vi "Planck-Curve-Sun-Earth.vi"() -> ()   [LabVIEW 2012]
panel:
  in  "Radius Sun (km)":dbl[unit]=696300.0
  in  "Distance Sun-Earth (km)":dbl[unit]=149600000.0
  out "Integral emittance (W m-2) 2":dbl[unit]=348.509952
  out "Integral emittance reaching Earth* (W m-2)":dbl[unit]=342.26526039686814
  out "Max emission (µm)":dbl=10.3525
  out "Max. emission (µm)":dbl=0.5016787815853236
  in  "Temperature of Earth (K)":dbl=280.0 step=10.0
  out "Planck Curves":T1(graph)=[{[{0.1, "Spectral emittance"=8.364960435276347e-211}, {0.19990000000000002, "Spectral emittance"=8.6959170545306e-101}, {0.2998, "Spectral emittance"=1.8099170209444927e-64}, {0.39970000000000006, "Spectral emittance"=1.7259097573278146e-46}, {0.49960000000000004, "Spectral emittance"=8.248773701500351e-36}, {0.5995, "Spectral emittance"=9.198523833864638e-29}, {0.6994, "Spectral emittance"=8.828454193587492e-24}, {0.7993, "Spectral emittance"=4.4031815212407465e-20}, {0.8992, "Spectral emittance"=3.0885678859060627e-17}, {0.9991, "Spectral emittance"=5.526298362014247e-15}, {1.099, "Spectral emittance"=3.679604984270012e-13}, {1.1989, "Spectral emittance"=1.1717326507920772e-11}, {1.2988000000000002, "Spectral emittance"=2.1218031119056521e-10}, {1.3987, "Spectral emittance"=2.4714773986706854e-09}, {1.4986000000000002, "Spectral emittance"=2.026296957778333e-08}, {1.5985, "Spectral emittance"=1.2507918319570943e-07}, {1.6984000000000001, "Spectral emittance"=6.119092116801698e-07}, {1.7983000000000002, "Spectral emittance"=2.4687793597519062e-06}, {1.8982, "Spectral emittance"=8.475417144153042e-06}, {1.9981000000000002, "Spectral emittance"=2.538389327407048e-05}, {2.098, "Spectral emittance"=6.767286542067558e-05}, {2.1979, "Spectral emittance"=0.00016325141397348066}, {2.2978, "Spectral emittance"=0.0003612038583115582}, {2.3977, "Spectral emittance"=0.0007412641406731495}, {2.4976000000000003, "Spectral emittance"=0.0014242855905207156}, {2.5975, "Spectral emittance"=0.002582637286474993}, {2.6974, "Spectral emittance"=0.004449293080124171}, {2.7973000000000003, "Spectral emittance"=0.007324416803243446}, {2.8972, "Spectral emittance"=0.011578470678244027}, {2.9971, "Spectral emittance"=0.01765123031017269}, {3.097, "Spectral emittance"=0.02604650857371942}, {3.1969000000000003, "Spectral emittance"=0.03732280325198327}, {3.2968, "Spectral emittance"=0.05208043469197373}, {3.3967, "Spectral emittance"=0.07094599565545717}, {3.4966000000000004, "Spectral emittance"=0.09455508234795544}, {3.5965000000000003, "Spectral emittance"=0.12353431695563427}, {3.6964, "Spectral emittance"=0.15848362355184462}, {3.7963, "Spectral emittance"=0.19995960311314315}, {3.8962000000000003, "Spectral emittance"=0.24846069362576262}, {3.9961, "Spectral emittance"=0.3044146203411553}, {4.096, "Spectral emittance"=0.3681684580016202}, {4.1959, "Spectral emittance"=0.43998145557952256}, {4.2958, "Spectral emittance"=0.520020624361168}, {4.3957, "Spectral emittance"=0.6083589674476632}, {4.4956, "Spectral emittance"=0.7049761348639901}, {4.5954999999999995, "Spectral emittance"=0.8097612227761682}, {4.695399999999999, "Spectral emittance"=0.922517395338843}, {4.7953, "Spectral emittance"=1.0429679898876865}, {4.8952, "Spectral emittance"=1.1707637665166895}, {4.9951, "Spectral emittance"=1.3054909774465249}, {5.095, "Spectral emittance"=1.4466799561417691}, {5.1949, "Spectral emittance"=1.5938139574417893}, {5.2947999999999995, "Spectral emittance"=1.746338015119278}, {5.394699999999999, "Spectral emittance"=1.9036676199059903}, {5.4946, "Spectral emittance"=2.0651970572888416}, {5.5945, "Spectral emittance"=2.2303072789255776}, {5.6944, "Spectral emittance"=2.398373213421066}, {5.7943, "Spectral emittance"=2.568770450857218}, {5.8942, "Spectral emittance"=2.7408812605796196}, {5.9940999999999995, "Spectral emittance"=2.9140999232282954}, {6.093999999999999, "Spectral emittance"=3.087837375939863}, {6.1939, "Spectral emittance"=3.2615251842392343}, {6.2938, "Spectral emittance"=3.434618865652263}, {6.3937, "Spectral emittance"=3.6066005988233463}, {6.4936, "Spectral emittance"=3.7769813582477663}, {6.5935, "Spectral emittance"=3.9453025189657405}, {6.6934, "Spectral emittance"=4.11113697803727}, {6.7932999999999995, "Spectral emittance"=4.274089840628593}, {6.8932, "Spectral emittance"=4.433798718369521}, {6.9931, "Spectral emittance"=4.589933686534616}, {7.093, "Spectral emittance"=4.742196944778176}, {7.1929, "Spectral emittance"=4.890322223801563}, {7.2928, "Spectral emittance"=5.034073977611674}, {7.3927, "Spectral emittance"=5.173246398075205}, {7.4925999999999995, "Spectral emittance"=5.307662285394177}, {7.5925, "Spectral emittance"=5.437171805013628}, {7.6924, "Spectral emittance"=5.561651158391748}, {7.7923, "Spectral emittance"=5.6810011920703}, {7.8922, "Spectral emittance"=5.795145966619549}, {7.9921, "Spectral emittance"=5.904031304325348}, {8.092, "Spectral emittance"=6.0076233319561565}, {8.1919, "Spectral emittance"=6.105907032605797}, {8.2918, "Spectral emittance"=6.198884818458783}, {8.3917, "Spectral emittance"=6.286575134369183}, {8.4916, "Spectral emittance"=6.3690111003778735}, {8.5915, "Spectral emittance"=6.446239199709471}, {8.6914, "Spectral emittance"=6.5183180173808895}, {8.7913, "Spectral emittance"=6.585317033308664}, {8.8912, "Spectral emittance"=6.647315472709573}, {8.9911, "Spectral emittance"=6.704401215638868}, {9.091, "Spectral emittance"=6.756669766689266}, {9.1909, "Spectral emittance"=6.804223285171723}, {9.290799999999999, "Spectral emittance"=6.8471696755032685}, {9.3907, "Spectral emittance"=6.885621737028204}, {9.4906, "Spectral emittance"=6.9196963720858555}, {9.5905, "Spectral emittance"=6.9495138508015994}, {9.6904, "Spectral emittance"=6.975197130808835}, {9.7903, "Spectral emittance"=6.996871229900023}, {9.8902, "Spectral emittance"=7.014662649447174}, {9.9901, "Spectral emittance"=7.0286988463194655}, {10.09, "Spectral emittance"=7.039107750951338}, {10.1899, "Spectral emittance"=7.046017329173741}, {10.2898, "Spectral emittance"=7.0495551854083}, {10.3897, "Spectral emittance"=7.049848204834858}, {10.4896, "Spectral emittance"=7.0470222321733305}, {10.5895, "Spectral emittance"=7.041201784767353}, {10.6894, "Spectral emittance"=7.032509797716861}, {10.7893, "Spectral emittance"=7.021067398876403}, {10.8892, "Spectral emittance"=7.006993711614304}, {10.9891, "Spectral emittance"=6.990405683311289}, {11.089, "Spectral emittance"=6.971417937665443}, {11.1889, "Spectral emittance"=6.95014264896128}, {11.2888, "Spectral emittance"=6.926689436552586}, {11.3887, "Spectral emittance"=6.90116527790176}, {11.4886, "Spectral emittance"=6.87367443861015}, {11.5885, "Spectral emittance"=6.844318417964861}, {11.6884, "Spectral emittance"=6.813195908616571}, {11.7883, "Spectral emittance"=6.780402769089453}, {11.8882, "Spectral emittance"=6.746032007908319}, {11.9881, "Spectral emittance"=6.710173778209088}, {12.088, "Spectral emittance"=6.672915381776411}, {12.1879, "Spectral emittance"=6.634341281526565}, {12.2878, "Spectral emittance"=6.5945331215249094}, {12.3877, "Spectral emittance"=6.553569753694313}, {12.4876, "Spectral emittance"=6.511527270435169}, {12.5875, "Spectral emittance"=6.468479042437906}, {12.6874, "Spectral emittance"=6.424495761025834}, {12.7873, "Spectral emittance"=6.37964548442006}, {12.8872, "Spectral emittance"=6.333993687368466}, {12.9871, "Spectral emittance"=6.287603313627812}, {13.087, "Spectral emittance"=6.240534830832629}, {13.1869, "Spectral emittance"=6.192846287325347}, {13.2868, "Spectral emittance"=6.144593370561008}, {13.3867, "Spectral emittance"=6.095829466735368}, {13.4866, "Spectral emittance"=6.046605721318699}, {13.5865, "Spectral emittance"=5.996971100208376}, {13.6864, "Spectral emittance"=5.9469724512419}, {13.7863, "Spectral emittance"=5.896654565838474}, {13.8862, "Spectral emittance"=5.846060240561751}, {13.9861, "Spectral emittance"=5.7952303384187465}, {14.086, "Spectral emittance"=5.744203849730753}, {14.1859, "Spectral emittance"=5.69301795243114}, {14.2858, "Spectral emittance"=5.641708071662418}, {14.3857, "Spectral emittance"=5.590307938560988}, {14.4856, "Spectral emittance"=5.538849648132664}, {14.5855, "Spectral emittance"=5.487363716135555}, {14.6854, "Spectral emittance"=5.435879134899017}, {14.7853, "Spectral emittance"=5.384423428018584}, {14.8852, "Spectral emittance"=5.333022703876983}, {14.9851, "Spectral emittance"=5.281701707950388}, {15.085, "Spectral emittance"=5.230483873867502}, {15.1849, "Spectral emittance"=5.179391373196531}, {15.2848, "Spectral emittance"=5.128445163941869}, {15.3847, "Spectral emittance"=5.0776650377384644}, {15.4846, "Spectral emittance"=5.027069665737203}, {15.5845, "Spectral emittance"=4.976676643179638}, {15.6844, "Spectral emittance"=4.926502532664633}, {15.7843, "Spectral emittance"=4.876562906113421}, {15.8842, "Spectral emittance"=4.826872385443039}, {15.9841, "Spectral emittance"=4.777444681960884}, {16.084, "Spectral emittance"=4.728292634496075}, {16.1839, "Spectral emittance"=4.679428246285375}, {16.283800000000003, "Spectral emittance"=4.630862720633445}, {16.3837, "Spectral emittance"=4.582606495368965}, {16.483600000000003, "Spectral emittance"=4.534669276119527}, {16.5835, "Spectral emittance"=4.487060068429441}, {16.683400000000002, "Spectral emittance"=4.4397872087455506}, {16.7833, "Spectral emittance"=4.39285839429704}, {16.883200000000002, "Spectral emittance"=4.346280711895674}, {16.9831, "Spectral emittance"=4.300060665683666}, {17.083000000000002, "Spectral emittance"=4.254204203856336}, {17.182900000000004, "Spectral emittance"=4.2087167443872815}, {17.2828, "Spectral emittance"=4.163603199783656}, {17.382700000000003, "Spectral emittance"=4.118868000899198}, {17.4826, "Spectral emittance"=4.074515119832661}, {17.582500000000003, "Spectral emittance"=4.030548091938943}, {17.6824, "Spectral emittance"=3.98697003698018}, {17.782300000000003, "Spectral emittance"=3.9437836794435865}, {17.8822, "Spectral emittance"=3.900991368052641}, {17.982100000000003, "Spectral emittance"=3.8585950944976277}, {18.082, "Spectral emittance"=3.8165965114113876}, {18.181900000000002, "Spectral emittance"=3.774996949615298}, {18.2818, "Spectral emittance"=3.7337974346603806}, {18.381700000000002, "Spectral emittance"=3.6929987026876168}, {18.4816, "Spectral emittance"=3.6526012156312277}, {18.581500000000002, "Spectral emittance"=3.6126051757879423}, {18.681400000000004, "Spectral emittance"=3.5730105397749043}, {18.7813, "Spectral emittance"=3.533817031898094}, {18.881200000000003, "Spectral emittance"=3.495024156952726}, {18.9811, "Spectral emittance"=3.4566312124764247}, {19.081000000000003, "Spectral emittance"=3.4186373004753765}, {19.1809, "Spectral emittance"=3.3810413386431777}, {19.280800000000003, "Spectral emittance"=3.343842071091367}, {19.3807, "Spectral emittance"=3.3070380786102116}, {19.480600000000003, "Spectral emittance"=3.2706277884776362}, {19.5805, "Spectral emittance"=3.234609483833671}, {19.680400000000002, "Spectral emittance"=3.198981312637236}, {19.7803, "Spectral emittance"=3.1637412962215428}, {19.880200000000002, "Spectral emittance"=3.1288873374638113}, {19.9801, "Spectral emittance"=3.094417228584553}, {20.080000000000002, "Spectral emittance"=3.0603286585910827}, {20.179900000000004, "Spectral emittance"=3.0266192203794744}, {20.2798, "Spectral emittance"=2.9932864175086373}, {20.379700000000003, "Spectral emittance"=2.960327670659748}, {20.4796, "Spectral emittance"=2.927740323793792}, {20.579500000000003, "Spectral emittance"=2.8955216500194996}, {20.6794, "Spectral emittance"=2.8636688571835296}, {20.779300000000003, "Spectral emittance"=2.8321790931943336}, {20.8792, "Spectral emittance"=2.801049451090704}, {20.979100000000003, "Spectral emittance"=2.770276973865575}, {21.079, "Spectral emittance"=2.739858659055311}, {21.178900000000002, "Spectral emittance"=2.709791463104285}, {21.2788, "Spectral emittance"=2.6800723055141966}, {21.378700000000002, "Spectral emittance"=2.650698072787203}, {21.478600000000004, "Spectral emittance"=2.6216656221716557}, {21.578500000000002, "Spectral emittance"=2.5929717852187655}, {21.678400000000003, "Spectral emittance"=2.5646133711583468}, {21.7783, "Spectral emittance"=2.536587170101388}, {21.878200000000003, "Spectral emittance"=2.508889956076877}, {21.9781, "Spectral emittance"=2.481518489910098}, {22.078000000000003, "Spectral emittance"=2.454469521949257}, {22.1779, "Spectral emittance"=2.4277397946470476}, {22.277800000000003, "Spectral emittance"=2.4013260450035308}, {22.3777, "Spectral emittance"=2.375225006876393}, {22.477600000000002, "Spectral emittance"=2.3494334131644634}, {22.5775, "Spectral emittance"=2.323947997870073}, {22.677400000000002, "Spectral emittance"=2.298765498045672}, {22.7773, "Spectral emittance"=2.2738826556298677}, {22.877200000000002, "Spectral emittance"=2.249296219177825}, {22.977100000000004, "Spectral emittance"=2.2250029454908007}, {23.077, "Spectral emittance"=2.200999601149372}, {23.176900000000003, "Spectral emittance"=2.177282963954719}, {23.2768, "Spectral emittance"=2.153849824282165}, {23.376700000000003, "Spectral emittance"=2.130696986350989}, {23.4766, "Spectral emittance"=2.107821269414365}, {23.576500000000003, "Spectral emittance"=2.0852195088730956}, {23.6764, "Spectral emittance"=2.0628885573167186}, {23.776300000000003, "Spectral emittance"=2.0408252854953273}, {23.8762, "Spectral emittance"=2.0190265832253917}, {23.976100000000002, "Spectral emittance"=1.997489360232653}, {24.076, "Spectral emittance"=1.9762105469350861}, {24.175900000000002, "Spectral emittance"=1.955187095168788}, {24.275800000000004, "Spectral emittance"=1.9344159788595012}, {24.375700000000002, "Spectral emittance"=1.9138941946423955}, {24.475600000000004, "Spectral emittance"=1.8936187624326093}, {24.5755, "Spectral emittance"=1.8735867259489465}, {24.675400000000003, "Spectral emittance"=1.8537951531930053}, {24.7753, "Spectral emittance"=1.8342411368859517}, {24.875200000000003, "Spectral emittance"=1.8149217948650154}, {24.9751, "Spectral emittance"=1.7958342704417296}, {25.075000000000003, "Spectral emittance"=1.7769757327238183}, {25.1749, "Spectral emittance"=1.7583433769025807}, {25.274800000000003, "Spectral emittance"=1.7399344245075181}, {25.3747, "Spectral emittance"=1.721746123629889}, {25.474600000000002, "Spectral emittance"=1.7037757491167793}, {25.5745, "Spectral emittance"=1.6860206027372513}, {25.674400000000002, "Spectral emittance"=1.6684780133220076}, {25.774300000000004, "Spectral emittance"=1.6511453368779851}, {25.874200000000002, "Spectral emittance"=1.6340199566792168}, {25.974100000000004, "Spectral emittance"=1.617099283335235}, {26.074, "Spectral emittance"=1.600380754838246}, {26.173900000000003, "Spectral emittance"=1.583861836590235}, {26.2738, "Spectral emittance"=1.5675400214111157}, {26.373700000000003, "Spectral emittance"=1.551412829528995}, {26.4736, "Spectral emittance"=1.5354778085535652}, {26.573500000000003, "Spectral emittance"=1.5197325334335838}, {26.6734, "Spectral emittance"=1.5041746063993908}, {26.773300000000003, "Spectral emittance"=1.4888016568913147}, {26.8732, "Spectral emittance"=1.4736113414748393}, {26.973100000000002, "Spectral emittance"=1.4586013437433045}, {27.073, "Spectral emittance"=1.443769374208949}, {27.172900000000002, "Spectral emittance"=1.4291131701829756}, {27.272800000000004, "Spectral emittance"=1.4146304956453781}, {27.372700000000002, "Spectral emittance"=1.400319141105174}, {27.472600000000003, "Spectral emittance"=1.386176923451676}, {27.5725, "Spectral emittance"=1.3722016857974078}, {27.672400000000003, "Spectral emittance"=1.358391297313249}, {27.7723, "Spectral emittance"=1.344743653056341}, {27.872200000000003, "Spectral emittance"=1.3312566737912725}, {27.9721, "Spectral emittance"=1.3179283058050717}, {28.072000000000003, "Spectral emittance"=1.3047565207164253}, {28.1719, "Spectral emittance"=1.2917393152796304}, {28.271800000000002, "Spectral emittance"=1.2788747111836607}, {28.3717, "Spectral emittance"=1.2661607548467768}, {28.471600000000002, "Spectral emittance"=1.2535955172070623}, {28.571500000000004, "Spectral emittance"=1.2411770935092539}, {28.671400000000002, "Spectral emittance"=1.228903603088199}, {28.771300000000004, "Spectral emittance"=1.216773189149305}, {28.8712, "Spectral emittance"=1.2047840185462593}, {28.971100000000003, "Spectral emittance"=1.1929342815563344}, {29.071, "Spectral emittance"=1.1812221916535715}, {29.170900000000003, "Spectral emittance"=1.169645985280084}, {29.2708, "Spectral emittance"=1.1582039216157645}, {29.370700000000003, "Spectral emittance"=1.1468942823466146}, {29.4706, "Spectral emittance"=1.1357153714319423}, {29.570500000000003, "Spectral emittance"=1.124665514870623}, {29.6704, "Spectral emittance"=1.1137430604666556}, {29.770300000000002, "Spectral emittance"=1.1029463775941764}, {29.8702, "Spectral emittance"=1.0922738569621453}, {29.970100000000002, "Spectral emittance"=1.0817239103788492}, {30.070000000000004, "Spectral emittance"=1.071294970516402}, {30.169900000000002, "Spectral emittance"=1.060985490675393}, {30.269800000000004, "Spectral emittance"=1.0507939445498173}, {30.3697, "Spectral emittance"=1.0407188259924443}, {30.469600000000003, "Spectral emittance"=1.0307586487807343}, {30.5695, "Spectral emittance"=1.0209119463834357}, {30.669400000000003, "Spectral emittance"=1.0111772717279688}, {30.7693, "Spectral emittance"=1.0015531969687084}, {30.869200000000003, "Spectral emittance"=0.9920383132562639}, {30.9691, "Spectral emittance"=0.9826312305078492}, {31.069000000000003, "Spectral emittance"=0.9733305771788243}, {31.1689, "Spectral emittance"=0.9641350000355086}, {31.268800000000002, "Spectral emittance"=0.955043163929317}, {31.368700000000004, "Spectral emittance"=0.9460537515723151}, {31.468600000000002, "Spectral emittance"=0.9371654633142374}, {31.568500000000004, "Spectral emittance"=0.9283770169210447}, {31.668400000000002, "Spectral emittance"=0.919687147355077}, {31.768300000000004, "Spectral emittance"=0.9110946065568404}, {31.8682, "Spectral emittance"=0.9025981632285007}, {31.968100000000003, "Spectral emittance"=0.8941966026190978}, {32.068, "Spectral emittance"=0.8858887263115556}, {32.1679, "Spectral emittance"=0.8776733520114945}, {32.2678, "Spectral emittance"=0.8695493133379031}, {32.3677, "Spectral emittance"=0.8615154596156859}, {32.467600000000004, "Spectral emittance"=0.8535706556701202}, {32.5675, "Spectral emittance"=0.8457137816232546}, {32.6674, "Spectral emittance"=0.8379437326922503}, {32.7673, "Spectral emittance"=0.8302594189897144}, {32.867200000000004, "Spectral emittance"=0.8226597653260169}, {32.9671, "Spectral emittance"=0.8151437110136212}, {33.067, "Spectral emittance"=0.807710209673436}, {33.166900000000005, "Spectral emittance"=0.800358229043198}, {33.2668, "Spectral emittance"=0.793086750787901}, {33.3667, "Spectral emittance"=0.785894770312271}, {33.4666, "Spectral emittance"=0.7787812965752925}, {33.566500000000005, "Spectral emittance"=0.7717453519067999}, {33.6664, "Spectral emittance"=0.7647859718261235}, {33.7663, "Spectral emittance"=0.7579022048627951}, {33.8662, "Spectral emittance"=0.7510931123793185}, {33.966100000000004, "Spectral emittance"=0.7443577683959898}, {34.066, "Spectral emittance"=0.7376952594177828}, {34.1659, "Spectral emittance"=0.7311046842632697}, {34.265800000000006, "Spectral emittance"=0.7245851538955962}, {34.365700000000004, "Spectral emittance"=0.7181357912554939}, {34.4656, "Spectral emittance"=0.711755731096313}, {34.5655, "Spectral emittance"=0.7054441198210865}, {34.665400000000005, "Spectral emittance"=0.6992001153215969}, {34.7653, "Spectral emittance"=0.693022886819455}, {34.8652, "Spectral emittance"=0.6869116147091548}, {34.9651, "Spectral emittance"=0.6808654904031197}, {35.065000000000005, "Spectral emittance"=0.6748837161787099}, {35.1649, "Spectral emittance"=0.6689655050271811}, {35.2648, "Spectral emittance"=0.6631100805045879}, {35.3647, "Spectral emittance"=0.6573166765846097}, {35.464600000000004, "Spectral emittance"=0.651584537513287}, {35.5645, "Spectral emittance"=0.6459129176656634}, {35.6644, "Spectral emittance"=0.6403010814042939}, {35.764300000000006, "Spectral emittance"=0.6347483029396324}, {35.864200000000004, "Spectral emittance"=0.6292538661922606}, {35.9641, "Spectral emittance"=0.6238170646569539}, {36.064, "Spectral emittance"=0.6184372012685628}, {36.163900000000005, "Spectral emittance"=0.613113588269693}, {36.2638, "Spectral emittance"=0.6078455470801709}, {36.3637, "Spectral emittance"=0.60263240816827}, {36.4636, "Spectral emittance"=0.5974735109236881}, {36.563500000000005, "Spectral emittance"=0.5923682035322556}, {36.6634, "Spectral emittance"=0.5873158428523532}, {36.7633, "Spectral emittance"=0.5823157942930236}, {36.8632, "Spectral emittance"=0.5773674316937631}, {36.963100000000004, "Spectral emittance"=0.5724701372059678}, {37.063, "Spectral emittance"=0.5676233011760222}, {37.1629, "Spectral emittance"=0.5628263220300073}, {37.262800000000006, "Spectral emittance"=0.558078606160014}, {37.362700000000004, "Spectral emittance"=0.5533795678120416}, {37.4626, "Spectral emittance"=0.548728628975461}, {37.5625, "Spectral emittance"=0.5441252192740305}, {37.662400000000005, "Spectral emittance"=0.5395687758584364}, {37.7623, "Spectral emittance"=0.5350587433003539}, {37.8622, "Spectral emittance"=0.530594573487991}, {37.9621, "Spectral emittance"=0.5261757255231181}, {38.062000000000005, "Spectral emittance"=0.5218016656195503}, {38.1619, "Spectral emittance"=0.5174718670030699}, {38.2618, "Spectral emittance"=0.5131858098127712}, {38.3617, "Spectral emittance"=0.5089429810038071}, {38.461600000000004, "Spectral emittance"=0.5047428742515269}, {38.5615, "Spectral emittance"=0.5005849898569754}, {38.6614, "Spectral emittance"=0.4964688346537483}, {38.761300000000006, "Spectral emittance"=0.4923939219161791}, {38.861200000000004, "Spectral emittance"=0.4883597712688397}, {38.9611, "Spectral emittance"=0.48436590859734435}, {39.061, "Spectral emittance"=0.48041186596043084}, {39.160900000000005, "Spectral emittance"=0.4764971815033076}, {39.2608, "Spectral emittance"=0.47262139937225234}, {39.3607, "Spectral emittance"=0.46878406963043395}, {39.4606, "Spectral emittance"=0.46498474817495794}, {39.560500000000005, "Spectral emittance"=0.46122299665510097}, {39.6604, "Spectral emittance"=0.45749838239173574}, {39.7603, "Spectral emittance"=0.453810478297916}, {39.8602, "Spectral emittance"=0.45015886280061135}, {39.960100000000004, "Spectral emittance"=0.44654311976358}, {40.06, "Spectral emittance"=0.4429628384113561}, {40.1599, "Spectral emittance"=0.4394176132543394}, {40.259800000000006, "Spectral emittance"=0.435907044014977}, {40.359700000000004, "Spectral emittance"=0.43243073555501105}, {40.4596, "Spectral emittance"=0.42898829780378817}, {40.5595, "Spectral emittance"=0.42557934568760947}, {40.659400000000005, "Spectral emittance"=0.4222034990601068}, {40.7593, "Spectral emittance"=0.4188603826336374}, {40.8592, "Spectral emittance"=0.41554962591166805}, {40.9591, "Spectral emittance"=0.41227086312215405}, {41.059000000000005, "Spectral emittance"=0.40902373315187923}, {41.1589, "Spectral emittance"=0.40580787948176095}, {41.2588, "Spectral emittance"=0.40262295012309046}, {41.358700000000006, "Spectral emittance"=0.3994685975547073}, {41.458600000000004, "Spectral emittance"=0.39634447866108924}, {41.5585, "Spectral emittance"=0.3932502546713411}, {41.6584, "Spectral emittance"=0.3901855910990786}, {41.758300000000006, "Spectral emittance"=0.3871501576831832}, {41.858200000000004, "Spectral emittance"=0.3841436283294271}, {41.9581, "Spectral emittance"=0.38116568105294346}, {42.058, "Spectral emittance"=0.3782159979215398}, {42.157900000000005, "Spectral emittance"=0.37529426499983665}, {42.2578, "Spectral emittance"=0.3724001722942203}, {42.3577, "Spectral emittance"=0.3695334136985988}, {42.4576, "Spectral emittance"=0.3666936869409494}, {42.557500000000005, "Spectral emittance"=0.36388069353064334}, {42.6574, "Spectral emittance"=0.3610941387065414}, {42.7573, "Spectral emittance"=0.35833373138584224}, {42.857200000000006, "Spectral emittance"=0.3555991841136789}, {42.957100000000004, "Spectral emittance"=0.35289021301344936}, {43.057, "Spectral emittance"=0.3502065377378676}, {43.1569, "Spectral emittance"=0.3475478814207316}, {43.256800000000005, "Spectral emittance"=0.3449139706293899}, {43.356700000000004, "Spectral emittance"=0.342304535317902}, {43.4566, "Spectral emittance"=0.3397193087808796}, {43.5565, "Spectral emittance"=0.33715802760799785}, {43.656400000000005, "Spectral emittance"=0.3346204316391704}, {43.7563, "Spectral emittance"=0.33210626392037373}, {43.8562, "Spectral emittance"=0.32961527066011354}, {43.9561, "Spectral emittance"=0.3271472011865251}, {44.056000000000004, "Spectral emittance"=0.32470180790509323}, {44.1559, "Spectral emittance"=0.32227884625698916}, {44.2558, "Spectral emittance"=0.319878074678008}, {44.355700000000006, "Spectral emittance"=0.3174992545581041}, {44.455600000000004, "Spectral emittance"=0.3151421502015131}, {44.5555, "Spectral emittance"=0.312806528787447}, {44.6554, "Spectral emittance"=0.3104921603313651}, {44.755300000000005, "Spectral emittance"=0.3081988176467983}, {44.8552, "Spectral emittance"=0.30592627630773067}, {44.9551, "Spectral emittance"=0.30367431461152156}, {45.055, "Spectral emittance"=0.3014427135423637}, {45.154900000000005, "Spectral emittance"=0.2992312567352701}, {45.2548, "Spectral emittance"=0.29703973044057963}, {45.3547, "Spectral emittance"=0.29486792348897367}, {45.4546, "Spectral emittance"=0.29271562725699707}, {45.554500000000004, "Spectral emittance"=0.2905826356330766}, {45.6544, "Spectral emittance"=0.2884687449840285}, {45.7543, "Spectral emittance"=0.2863737541220449}, {45.854200000000006, "Spectral emittance"=0.28429746427215835}, {45.954100000000004, "Spectral emittance"=0.28223967904017194}, {46.054, "Spectral emittance"=0.28020020438104826}, {46.1539, "Spectral emittance"=0.27817884856775515}, {46.253800000000005, "Spectral emittance"=0.27617542216055435}, {46.3537, "Spectral emittance"=0.2741897379767331}, {46.4536, "Spectral emittance"=0.27222161106076614}, {46.5535, "Spectral emittance"=0.27027085865490696}, {46.653400000000005, "Spectral emittance"=0.2683373001701972}, {46.7533, "Spectral emittance"=0.26642075715789165}, {46.8532, "Spectral emittance"=0.2645210532812902}, {46.9531, "Spectral emittance"=0.262638014287971}, {47.053000000000004, "Spectral emittance"=0.2607714679824202}, {47.1529, "Spectral emittance"=0.2589212441990513}, {47.2528, "Spectral emittance"=0.25708717477560716}, {47.352700000000006, "Spectral emittance"=0.255269093526941}, {47.452600000000004, "Spectral emittance"=0.2534668362191695}, {47.5525, "Spectral emittance"=0.25168024054419347}, {47.6524, "Spectral emittance"=0.24990914609457773}, {47.752300000000005, "Spectral emittance"=0.24815339433878875}, {47.8522, "Spectral emittance"=0.2464128285967832}, {47.9521, "Spectral emittance"=0.244687294015939}, {48.052, "Spectral emittance"=0.24297663754732968}, {48.151900000000005, "Spectral emittance"=0.2412807079223317}, {48.2518, "Spectral emittance"=0.2395993556295623}, {48.3517, "Spectral emittance"=0.2379324328921432}, {48.451600000000006, "Spectral emittance"=0.2362797936452824}, {48.551500000000004, "Spectral emittance"=0.2346412935141747}, {48.6514, "Spectral emittance"=0.23301678979220894}, {48.7513, "Spectral emittance"=0.23140614141948415}, {48.851200000000006, "Spectral emittance"=0.22980920896162707}, {48.951100000000004, "Spectral emittance"=0.2282258545889042}, {49.051, "Spectral emittance"=0.22665594205563008}, {49.1509, "Spectral emittance"=0.22509933667985974}, {49.250800000000005, "Spectral emittance"=0.22355590532336791}, {49.3507, "Spectral emittance"=0.222025516371908}, {49.4506, "Spectral emittance"=0.22050803971574381}, {49.5505, "Spectral emittance"=0.21900334673045532}, {49.650400000000005, "Spectral emittance"=0.21751131025801088}, {49.7503, "Spectral emittance"=0.21603180458810256}, {49.8502, "Spectral emittance"=0.21456470543974152}, {49.950100000000006, "Spectral emittance"=0.21310988994310828}, {50.050000000000004, "Spectral emittance"=0.211667236621656}, {50.1499, "Spectral emittance"=0.21023662537445972}, {50.2498, "Spectral emittance"=0.20881793745881247}, {50.349700000000006, "Spectral emittance"=0.2074110554730607}, {50.449600000000004, "Spectral emittance"=0.20601586333967747}, {50.5495, "Spectral emittance"=0.2046322462885687}, {50.6494, "Spectral emittance"=0.20326009084061042}, {50.749300000000005, "Spectral emittance"=0.20189928479141261}, {50.8492, "Spectral emittance"=0.20054971719530676}, {50.9491, "Spectral emittance"=0.19921127834955296}, {51.049, "Spectral emittance"=0.19788385977876477}, {51.148900000000005, "Spectral emittance"=0.19656735421954707}, {51.2488, "Spectral emittance"=0.19526165560534575}, {51.3487, "Spectral emittance"=0.19396665905150337}, {51.448600000000006, "Spectral emittance"=0.19268226084052006}, {51.548500000000004, "Spectral emittance"=0.19140835840751702}, {51.6484, "Spectral emittance"=0.19014485032589562}, {51.7483, "Spectral emittance"=0.18889163629319516}, {51.848200000000006, "Spectral emittance"=0.1876486171171417}, {51.948100000000004, "Spectral emittance"=0.18641569470188693}, {52.048, "Spectral emittance"=0.18519277203443496}, {52.1479, "Spectral emittance"=0.18397975317125206}, {52.247800000000005, "Spectral emittance"=0.1827765432250599}, {52.3477, "Spectral emittance"=0.18158304835180622}, {52.4476, "Spectral emittance"=0.1803991757378129}, {52.5475, "Spectral emittance"=0.17922483358709765}, {52.647400000000005, "Spectral emittance"=0.1780599311088664}, {52.7473, "Spectral emittance"=0.17690437850517624}, {52.8472, "Spectral emittance"=0.17575808695876238}, {52.947100000000006, "Spectral emittance"=0.1746209686210306}, {53.047000000000004, "Spectral emittance"=0.1734929366002116}, {53.1469, "Spectral emittance"=0.17237390494967295}, {53.2468, "Spectral emittance"=0.17126378865638942}, {53.346700000000006, "Spectral emittance"=0.17016250362956747}, {53.446600000000004, "Spectral emittance"=0.16906996668942217}, {53.5465, "Spectral emittance"=0.16798609555610405}, {53.6464, "Spectral emittance"=0.1669108088387742}, {53.746300000000005, "Spectral emittance"=0.16584402602482562}, {53.8462, "Spectral emittance"=0.16478566746924808}, {53.9461, "Spectral emittance"=0.1637356543841344}, {54.046, "Spectral emittance"=0.1626939088283265}, {54.145900000000005, "Spectral emittance"=0.16166035369719964}, {54.2458, "Spectral emittance"=0.16063491271258232}, {54.3457, "Spectral emittance"=0.15961751041280872}, {54.445600000000006, "Spectral emittance"=0.1586080721429045}, {54.545500000000004, "Spectral emittance"=0.15760652404490205}, {54.6454, "Spectral emittance"=0.15661279304828296}, {54.7453, "Spectral emittance"=0.15562680686054803}, {54.845200000000006, "Spectral emittance"=0.1546484939579109}, {54.945100000000004, "Spectral emittance"=0.1536777835761148}, {55.045, "Spectral emittance"=0.15271460570136944}, {55.1449, "Spectral emittance"=0.15175889106140794}, {55.244800000000005, "Spectral emittance"=0.1508105711166612}, {55.3447, "Spectral emittance"=0.1498695780515473}, {55.4446, "Spectral emittance"=0.14893584476587585}, {55.544500000000006, "Spectral emittance"=0.1480093048663645}, {55.644400000000005, "Spectral emittance"=0.14708989265826658}, {55.7443, "Spectral emittance"=0.14617754313710818}, {55.8442, "Spectral emittance"=0.14527219198053262}, {55.944100000000006, "Spectral emittance"=0.14437377554025158}, {56.044000000000004, "Spectral emittance"=0.1434822308341016}, {56.1439, "Spectral emittance"=0.14259749553820206}, {56.2438, "Spectral emittance"=0.14171950797921748}, {56.343700000000005, "Spectral emittance"=0.14084820712671806}, {56.4436, "Spectral emittance"=0.1399835325856411}, {56.5435, "Spectral emittance"=0.13912542458884802}, {56.6434, "Spectral emittance"=0.13827382398977958}, {56.743300000000005, "Spectral emittance"=0.13742867225520466}, {56.8432, "Spectral emittance"=0.13658991145806348}, {56.9431, "Spectral emittance"=0.1357574842704022}, {57.043000000000006, "Spectral emittance"=0.13493133395639906}, {57.142900000000004, "Spectral emittance"=0.13411140436548052}, {57.2428, "Spectral emittance"=0.1332976399255247}, {57.3427, "Spectral emittance"=0.13248998563615316}, {57.442600000000006, "Spectral emittance"=0.13168838706210823}, {57.542500000000004, "Spectral emittance"=0.13089279032671478}, {57.6424, "Spectral emittance"=0.13010314210542653}, {57.7423, "Spectral emittance"=0.1293193896194534}, {57.842200000000005, "Spectral emittance"=0.12854148062947146}, {57.9421, "Spectral emittance"=0.12776936342941278}, {58.042, "Spectral emittance"=0.12700298684033337}, {58.1419, "Spectral emittance"=0.12624230020436042}, {58.241800000000005, "Spectral emittance"=0.12548725337871552}, {58.3417, "Spectral emittance"=0.12473779672981405}, {58.4416, "Spectral emittance"=0.12399388112743943}, {58.541500000000006, "Spectral emittance"=0.12325545793899063}, {58.641400000000004, "Spectral emittance"=0.12252247902380331}, {58.7413, "Spectral emittance"=0.12179489672754137}, {58.8412, "Spectral emittance"=0.12107266387666049}, {58.941100000000006, "Spectral emittance"=0.12035573377294084}, {59.041000000000004, "Spectral emittance"=0.11964406018808872}, {59.1409, "Spectral emittance"=0.11893759735840588}, {59.2408, "Spectral emittance"=0.11823629997952596}, {59.340700000000005, "Spectral emittance"=0.1175401232012169}, {59.4406, "Spectral emittance"=0.11684902262224883}, {59.5405, "Spectral emittance"=0.11616295428532517}, {59.6404, "Spectral emittance"=0.11548187467207838}, {59.740300000000005, "Spectral emittance"=0.11480574069812707}, {59.8402, "Spectral emittance"=0.11413450970819593}, {59.9401, "Spectral emittance"=0.11346813947129473}, {60.040000000000006, "Spectral emittance"=0.11280658817595916}, {60.139900000000004, "Spectral emittance"=0.11214981442555012}, {60.2398, "Spectral emittance"=0.11149777723361029}, {60.3397, "Spectral emittance"=0.1108504360192803}, {60.439600000000006, "Spectral emittance"=0.11020775060276987}, {60.539500000000004, "Spectral emittance"=0.10956968120088614}, {60.6394, "Spectral emittance"=0.10893618842261668}, {60.7393, "Spectral emittance"=0.10830723326476718}, {60.839200000000005, "Spectral emittance"=0.1076827771076529}, {60.9391, "Spectral emittance"=0.10706278171084327}, {61.039, "Spectral emittance"=0.1064472092089587}, {61.1389, "Spectral emittance"=0.10583602210751905}, {61.238800000000005, "Spectral emittance"=0.1052291832788435}, {61.3387, "Spectral emittance"=0.10462665595799951}, {61.4386, "Spectral emittance"=0.10402840373880318}, {61.538500000000006, "Spectral emittance"=0.10343439056986643}, {61.638400000000004, "Spectral emittance"=0.10284458075069423}, {61.7383, "Spectral emittance"=0.10225893892782895}, {61.8382, "Spectral emittance"=0.10167743009104069}, {61.938100000000006, "Spectral emittance"=0.10110001956956563}, {62.038000000000004, "Spectral emittance"=0.10052667302838916}, {62.1379, "Spectral emittance"=0.09995735646457396}, {62.2378, "Spectral emittance"=0.09939203620363331}, {62.337700000000005, "Spectral emittance"=0.09883067889594799}, {62.4376, "Spectral emittance"=0.09827325151322684}, {62.5375, "Spectral emittance"=0.09771972134500932}, {62.63740000000001, "Spectral emittance"=0.0971700559952114}, {62.737300000000005, "Spectral emittance"=0.09662422337871235}, {62.8372, "Spectral emittance"=0.09608219171798296}, {62.9371, "Spectral emittance"=0.0955439295397545}, {63.037000000000006, "Spectral emittance"=0.095009405671727}, {63.136900000000004, "Spectral emittance"=0.09447858923931803}, {63.2368, "Spectral emittance"=0.09395144966245007}, {63.3367, "Spectral emittance"=0.09342795665237602}, {63.436600000000006, "Spectral emittance"=0.09290808020854296}, {63.536500000000004, "Spectral emittance"=0.09239179061549418}, {63.6364, "Spectral emittance"=0.09187905843980648}, {63.7363, "Spectral emittance"=0.09136985452706566}, {63.836200000000005, "Spectral emittance"=0.09086414999887711}, {63.9361, "Spectral emittance"=0.09036191624991242}, {64.036, "Spectral emittance"=0.08986312494499078}, {64.13589999999999, "Spectral emittance"=0.08936774801619522}, {64.2358, "Spectral emittance"=0.08887575766002281}, {64.3357, "Spectral emittance"=0.08838712633456917}, {64.4356, "Spectral emittance"=0.08790182675674575}, {64.5355, "Spectral emittance"=0.08741983189952983}, {64.63539999999999, "Spectral emittance"=0.0869411149892481}, {64.7353, "Spectral emittance"=0.08646564950289072}, {64.8352, "Spectral emittance"=0.08599340916545818}, {64.93509999999999, "Spectral emittance"=0.08552436794733904}, {65.035, "Spectral emittance"=0.08505850006171826}, {65.1349, "Spectral emittance"=0.08459577996201628}, {65.23479999999999, "Spectral emittance"=0.08413618233935773}, {65.3347, "Spectral emittance"=0.08367968212007021}, {65.43459999999999, "Spectral emittance"=0.08322625446321241}, {65.5345, "Spectral emittance"=0.08277587475813016}, {65.6344, "Spectral emittance"=0.08232851862204234}, {65.73429999999999, "Spectral emittance"=0.08188416189765421}, {65.8342, "Spectral emittance"=0.08144278065079803}, {65.9341, "Spectral emittance"=0.0810043511681025}, {66.03399999999999, "Spectral emittance"=0.08056884995468815}, {66.1339, "Spectral emittance"=0.08013625373188966}, {66.2338, "Spectral emittance"=0.07970653943500482}, {66.3337, "Spectral emittance"=0.07927968421106983}, {66.4336, "Spectral emittance"=0.0788556654166594}, {66.53349999999999, "Spectral emittance"=0.07843446061571327}, {66.6334, "Spectral emittance"=0.07801604757738712}, {66.7333, "Spectral emittance"=0.07760040427392903}, {66.83319999999999, "Spectral emittance"=0.07718750887857899}, {66.9331, "Spectral emittance"=0.07677733976349428}, {67.033, "Spectral emittance"=0.07636987549769753}, {67.13289999999999, "Spectral emittance"=0.07596509484504876}, {67.2328, "Spectral emittance"=0.07556297676224014}, {67.3327, "Spectral emittance"=0.07516350039681494}, {67.4326, "Spectral emittance"=0.07476664508520768}, {67.5325, "Spectral emittance"=0.07437239035080734}, {67.63239999999999, "Spectral emittance"=0.07398071590204315}, {67.7323, "Spectral emittance"=0.07359160163049125}, {67.8322, "Spectral emittance"=0.07320502760900328}, {67.93209999999999, "Spectral emittance"=0.07282097408985691}, {68.032, "Spectral emittance"=0.07243942150292614}, {68.1319, "Spectral emittance"=0.07206035045387342}, {68.23179999999999, "Spectral emittance"=0.0716837417223617}, {68.3317, "Spectral emittance"=0.0713095762602868}, {68.4316, "Spectral emittance"=0.07093783519003025}, {68.5315, "Spectral emittance"=0.07056849980273094}, {68.6314, "Spectral emittance"=0.0702015515565771}, {68.73129999999999, "Spectral emittance"=0.0698369720751173}, {68.8312, "Spectral emittance"=0.0694747431455902}, {68.9311, "Spectral emittance"=0.0691148467172732}, {69.03099999999999, "Spectral emittance"=0.06875726489985018}, {69.1309, "Spectral emittance"=0.06840197996179662}, {69.2308, "Spectral emittance"=0.06804897432878336}, {69.3307, "Spectral emittance"=0.06769823058209856}, {69.4306, "Spectral emittance"=0.06734973145708638}, {69.53049999999999, "Spectral emittance"=0.067003459841604}, {69.6304, "Spectral emittance"=0.06665939877449521}, {69.7303, "Spectral emittance"=0.06631753144408174}, {69.83019999999999, "Spectral emittance"=0.06597784118667051}, {69.9301, "Spectral emittance"=0.06564031148507794}, {70.03, "Spectral emittance"=0.06530492596717093}, {70.12989999999999, "Spectral emittance"=0.06497166840442352}, {70.2298, "Spectral emittance"=0.06464052271048963}, {70.3297, "Spectral emittance"=0.06431147293979206}, {70.4296, "Spectral emittance"=0.06398450328612652}, {70.5295, "Spectral emittance"=0.06365959808128127}, {70.62939999999999, "Spectral emittance"=0.06333674179367234}, {70.7293, "Spectral emittance"=0.06301591902699313}, {70.8292, "Spectral emittance"=0.06269711451887965}, {70.92909999999999, "Spectral emittance"=0.06238031313958967}, {71.029, "Spectral emittance"=0.06206549989069684}, {71.1289, "Spectral emittance"=0.06175265990379938}, {71.22879999999999, "Spectral emittance"=0.0614417784392421}, {71.3287, "Spectral emittance"=0.061132840884853205}, {71.4286, "Spectral emittance"=0.06082583275469466}, {71.5285, "Spectral emittance"=0.06052073968782611}, {71.6284, "Spectral emittance"=0.060217547447082014}, {71.72829999999999, "Spectral emittance"=0.0599162419178632}, {71.8282, "Spectral emittance"=0.059616809106940054}, {71.9281, "Spectral emittance"=0.05931923514126997}, {72.02799999999999, "Spectral emittance"=0.05902350626682717}, {72.1279, "Spectral emittance"=0.058729608847444936}, {72.2278, "Spectral emittance"=0.05843752936367095}, {72.3277, "Spectral emittance"=0.058147254411634854}, {72.4276, "Spectral emittance"=0.05785877070192761}, {72.52749999999999, "Spectral emittance"=0.0575720650584939}, {72.6274, "Spectral emittance"=0.05728712441753534}, {72.7273, "Spectral emittance"=0.057003935826426516}, {72.82719999999999, "Spectral emittance"=0.056722486442642335}, {72.9271, "Spectral emittance"=0.05644276353269637}, {73.027, "Spectral emittance"=0.05616475447109175}, {73.12689999999999, "Spectral emittance"=0.05588844673928242}, {73.2268, "Spectral emittance"=0.055613827924645476}, {73.3267, "Spectral emittance"=0.05534088571946548}, {73.4266, "Spectral emittance"=0.05506960791992855}, {73.5265, "Spectral emittance"=0.05479998242512773}, {73.62639999999999, "Spectral emittance"=0.05453199723607906}, {73.7263, "Spectral emittance"=0.05426564045474771}, {73.8262, "Spectral emittance"=0.05400090028308521}, {73.92609999999999, "Spectral emittance"=0.053737765022075966}, {74.026, "Spectral emittance"=0.053476223070794804}, {74.1259, "Spectral emittance"=0.05321626292547404}, {74.22579999999999, "Spectral emittance"=0.0529578731785806}, {74.3257, "Spectral emittance"=0.052701042517902634}, {74.4256, "Spectral emittance"=0.052445759725646475}, {74.5255, "Spectral emittance"=0.05219201367754245}, {74.6254, "Spectral emittance"=0.05193979334196027}, {74.72529999999999, "Spectral emittance"=0.05168908777903432}, {74.8252, "Spectral emittance"=0.051439886139797296}, {74.9251, "Spectral emittance"=0.05119217766532359}, {75.02499999999999, "Spectral emittance"=0.05094595168588174}, {75.1249, "Spectral emittance"=0.05070119762009497}, {75.2248, "Spectral emittance"=0.05045790497411175}, {75.32469999999999, "Spectral emittance"=0.05021606334078391}, {75.4246, "Spectral emittance"=0.049975662398854225}, {75.5245, "Spectral emittance"=0.04973669191215196}, {75.6244, "Spectral emittance"=0.04949914172879701}, {75.7243, "Spectral emittance"=0.04926300178041242}, {75.82419999999999, "Spectral emittance"=0.049028262081345066}, {75.9241, "Spectral emittance"=0.0487949127278942}, {76.024, "Spectral emittance"=0.04856294389754852}, {76.12389999999999, "Spectral emittance"=0.04833234584823092}, {76.2238, "Spectral emittance"=0.04810310891755073}, {76.3237, "Spectral emittance"=0.047875223522064345}, {76.4236, "Spectral emittance"=0.047648680156543194}, {76.5235, "Spectral emittance"=0.0474234693932492}, {76.62339999999999, "Spectral emittance"=0.047199581881217895}, {76.7233, "Spectral emittance"=0.04697700834554881}, {76.8232, "Spectral emittance"=0.04675573958670348}, {76.92309999999999, "Spectral emittance"=0.0465357664798102}, {77.023, "Spectral emittance"=0.04631707997397632}, {77.1229, "Spectral emittance"=0.04609967109160758}, {77.22279999999999, "Spectral emittance"=0.045883530927734215}, {77.3227, "Spectral emittance"=0.04566865064934414}, {77.4226, "Spectral emittance"=0.045455021494723045}, {77.5225, "Spectral emittance"=0.04524263477280115}, {77.6224, "Spectral emittance"=0.045031481862506384}, {77.72229999999999, "Spectral emittance"=0.04482155421212483}, {77.8222, "Spectral emittance"=0.04461284333866701}, {77.9221, "Spectral emittance"=0.044405340827241124}, {78.02199999999999, "Spectral emittance"=0.04419903833043227}, {78.1219, "Spectral emittance"=0.04399392756768832}, {78.2218, "Spectral emittance"=0.043790000324712024}, {78.32169999999999, "Spectral emittance"=0.04358724845285889}, {78.4216, "Spectral emittance"=0.04338566386854161}, {78.5215, "Spectral emittance"=0.04318523855264053}, {78.6214, "Spectral emittance"=0.04298596454991954}, {78.7213, "Spectral emittance"=0.04278783396844859}, {78.82119999999999, "Spectral emittance"=0.0425908389790316}, {78.9211, "Spectral emittance"=0.042394971814640206}, {79.021, "Spectral emittance"=0.042200224769853294}, {79.12089999999999, "Spectral emittance"=0.04200659020030216}, {79.2208, "Spectral emittance"=0.0418140605221212}, {79.3207, "Spectral emittance"=0.04162262821140416}, {79.4206, "Spectral emittance"=0.04143228580366591}, {79.5205, "Spectral emittance"=0.04124302589330944}, {79.62039999999999, "Spectral emittance"=0.04105484113309837}, {79.7203, "Spectral emittance"=0.04086772423363461}, {79.8202, "Spectral emittance"=0.040681667962841395}, {79.92009999999999, "Spectral emittance"=0.04049666514545146}, {80.02, "Spectral emittance"=0.040312708662499884}, {80.1199, "Spectral emittance"=0.04012979145082281}, {80.21979999999999, "Spectral emittance"=0.0399479065025605}, {80.3197, "Spectral emittance"=0.03976704686466546}, {80.4196, "Spectral emittance"=0.03958720563841564}, {80.5195, "Spectral emittance"=0.03940837597893245}, {80.6194, "Spectral emittance"=0.03923055109470318}, {80.71929999999999, "Spectral emittance"=0.03905372424710873}, {80.8192, "Spectral emittance"=0.03887788874995549}, {80.9191, "Spectral emittance"=0.038703037969012234}, {81.01899999999999, "Spectral emittance"=0.03852916532155134}, {81.1189, "Spectral emittance"=0.03835626427589457}, {81.2188, "Spectral emittance"=0.0381843283509636}, {81.31869999999999, "Spectral emittance"=0.038013351115834426}, {81.4186, "Spectral emittance"=0.03784332618929673}, {81.5185, "Spectral emittance"=0.03767424723941726}, {81.6184, "Spectral emittance"=0.03750610798310758}, {81.7183, "Spectral emittance"=0.03733890218569581}, {81.81819999999999, "Spectral emittance"=0.03717262366050321}, {81.9181, "Spectral emittance"=0.037007266268424106}, {82.018, "Spectral emittance"=0.03684282391751045}, {82.11789999999999, "Spectral emittance"=0.036679290562560356}, {82.2178, "Spectral emittance"=0.0365166602047104}, {82.3177, "Spectral emittance"=0.03635492689103226}, {82.4176, "Spectral emittance"=0.03619408471413295}, {82.5175, "Spectral emittance"=0.03603412781175915}, {82.6174, "Spectral emittance"=0.03587505036640538}, {82.7173, "Spectral emittance"=0.03571684660492573}, {82.8172, "Spectral emittance"=0.0355595107981497}, {82.91709999999999, "Spectral emittance"=0.03540303726050165}, {83.017, "Spectral emittance"=0.03524742034962355}, {83.1169, "Spectral emittance"=0.03509265446600214}, {83.21679999999999, "Spectral emittance"=0.034938734052599035}, {83.3167, "Spectral emittance"=0.03478565359448447}, {83.4166, "Spectral emittance"=0.03463340761847504}, {83.5165, "Spectral emittance"=0.03448199069277446}, {83.6164, "Spectral emittance"=0.034331397426617866}, {83.71629999999999, "Spectral emittance"=0.03418162246991966}, {83.8162, "Spectral emittance"=0.03403266051292473}, {83.9161, "Spectral emittance"=0.033884506285862884}, {84.01599999999999, "Spectral emittance"=0.033737154558606694}, {84.1159, "Spectral emittance"=0.033590600140332535}, {84.2158, "Spectral emittance"=0.033444837879185015}, {84.31569999999999, "Spectral emittance"=0.03329986266194449}, {84.4156, "Spectral emittance"=0.03315566941369764}, {84.5155, "Spectral emittance"=0.03301225309751149}, {84.6154, "Spectral emittance"=0.03286960871411032}, {84.7153, "Spectral emittance"=0.03272773130155556}, {84.81519999999999, "Spectral emittance"=0.03258661593492904}, {84.9151, "Spectral emittance"=0.03244625772601895}, {85.015, "Spectral emittance"=0.03230665182300889}, {85.11489999999999, "Spectral emittance"=0.03216779341016999}, {85.2148, "Spectral emittance"=0.03202967770755561}, {85.3147, "Spectral emittance"=0.03189229997069935}, {85.4146, "Spectral emittance"=0.03175565549031556}, {85.5145, "Spectral emittance"=0.03161973959200285}, {85.6144, "Spectral emittance"=0.03148454763595044}, {85.7143, "Spectral emittance"=0.031350075016647036}, {85.8142, "Spectral emittance"=0.03121631716259276}, {85.91409999999999, "Spectral emittance"=0.0310832695360136}, {86.014, "Spectral emittance"=0.030950927632578413}, {86.1139, "Spectral emittance"=0.03081928698111902}, {86.21379999999999, "Spectral emittance"=0.030688343143352465}, {86.3137, "Spectral emittance"=0.03055809171360604}, {86.4136, "Spectral emittance"=0.030428528318544996}, {86.5135, "Spectral emittance"=0.030299648616902673}, {86.6134, "Spectral emittance"=0.030171448299213144}, {86.71329999999999, "Spectral emittance"=0.030043923087546377}, {86.8132, "Spectral emittance"=0.029917068735245925}, {86.9131, "Spectral emittance"=0.029790881026668985}, {87.01299999999999, "Spectral emittance"=0.029665355776928918}, {87.1129, "Spectral emittance"=0.02954048883163997}, {87.2128, "Spectral emittance"=0.029416276066664797}, {87.31269999999999, "Spectral emittance"=0.029292713387863913}, {87.4126, "Spectral emittance"=0.029169796730847505}, {87.5125, "Spectral emittance"=0.029047522060729858}, {87.6124, "Spectral emittance"=0.028925885371885774}, {87.7123, "Spectral emittance"=0.02880488268770911}, {87.81219999999999, "Spectral emittance"=0.028684510060374053}, {87.9121, "Spectral emittance"=0.028564763570598038}, {88.012, "Spectral emittance"=0.02844563932740722}, {88.11189999999999, "Spectral emittance"=0.02832713346790388}, {88.2118, "Spectral emittance"=0.028209242157036147}, {88.3117, "Spectral emittance"=0.028091961587369707}, {88.41159999999999, "Spectral emittance"=0.02797528797886164}, {88.5115, "Spectral emittance"=0.027859217578636346}, {88.6114, "Spectral emittance"=0.027743746660763548}, {88.7113, "Spectral emittance"=0.027628871526038237}, {88.8112, "Spectral emittance"=0.027514588501762704}, {88.91109999999999, "Spectral emittance"=0.027400893941530557}, {89.011, "Spectral emittance"=0.027287784225012657}, {89.1109, "Spectral emittance"=0.027175255757745053}, {89.21079999999999, "Spectral emittance"=0.027063304970918838}, {89.3107, "Spectral emittance"=0.02695192832117188}, {89.4106, "Spectral emittance"=0.026841122290382494}, {89.5105, "Spectral emittance"=0.02673088338546497}, {89.6104, "Spectral emittance"=0.026621208138166944}, {89.7103, "Spectral emittance"=0.02651209310486859}, {89.8102, "Spectral emittance"=0.02640353486638367}, {89.9101, "Spectral emittance"=0.026295530027762384}, {90.00999999999999, "Spectral emittance"=0.02618807521809593}, {90.1099, "Spectral emittance"=0.026081167090322863}, {90.2098, "Spectral emittance"=0.02597480232103729}, {90.30969999999999, "Spectral emittance"=0.025868977610298712}, {90.4096, "Spectral emittance"=0.0257636896814434}, {90.5095, "Spectral emittance"=0.02565893528089793}, {90.6094, "Spectral emittance"=0.025554711177993898}, {90.7093, "Spectral emittance"=0.025451014164784545}, {90.80919999999999, "Spectral emittance"=0.02534784105586307}, {90.9091, "Spectral emittance"=0.02524518868818237}, {91.009, "Spectral emittance"=0.02514305392087663}, {91.10889999999999, "Spectral emittance"=0.0250414336350843}, {91.2088, "Spectral emittance"=0.024940324733772765}, {91.3087, "Spectral emittance"=0.024839724141564563}, {91.40859999999999, "Spectral emittance"=0.02473962880456514}, {91.5085, "Spectral emittance"=0.024640035690192127}, {91.6084, "Spectral emittance"=0.024540941787006193}, {91.7083, "Spectral emittance"=0.02444234410454335}, {91.8082, "Spectral emittance"=0.024344239673148627}, {91.90809999999999, "Spectral emittance"=0.024246625543811563}, {92.008, "Spectral emittance"=0.02414949878800279}, {92.1079, "Spectral emittance"=0.02405285649751224}, {92.20779999999999, "Spectral emittance"=0.023956695784288832}, {92.3077, "Spectral emittance"=0.023861013780281402}, {92.4076, "Spectral emittance"=0.023765807637281183}, {92.5075, "Spectral emittance"=0.023671074526765656}, {92.6074, "Spectral emittance"=0.02357681163974369}, {92.7073, "Spectral emittance"=0.023483016186602156}, {92.8072, "Spectral emittance"=0.023389685396953807}, {92.9071, "Spectral emittance"=0.023296816519486514}, {93.00699999999999, "Spectral emittance"=0.023204406821813923}, {93.1069, "Spectral emittance"=0.023112453590327195}, {93.2068, "Spectral emittance"=0.02302095413004833}, {93.30669999999999, "Spectral emittance"=0.022929905764484546}, {93.4066, "Spectral emittance"=0.022839305835484037}, {93.5065, "Spectral emittance"=0.022749151703092968}, {93.6064, "Spectral emittance"=0.02265944074541374}, {93.7063, "Spectral emittance"=0.022570170358464463}, {93.80619999999999, "Spectral emittance"=0.022481337956039668}, {93.9061, "Spectral emittance"=0.022392940969572173}, {94.006, "Spectral emittance"=0.022304976847996347}, {94.10589999999999, "Spectral emittance"=0.02221744305761226}, {94.2058, "Spectral emittance"=0.022130337081951237}, {94.3057, "Spectral emittance"=0.022043656421642552}, {94.40559999999999, "Spectral emittance"=0.02195739859428122}, {94.5055, "Spectral emittance"=0.02187156113429686}, {94.6054, "Spectral emittance"=0.021786141592823917}, {94.7053, "Spectral emittance"=0.021701137537572846}, {94.8052, "Spectral emittance"=0.021616546552702322}, {94.90509999999999, "Spectral emittance"=0.021532366238692834}, {95.005, "Spectral emittance"=0.02144859421222105}, {95.1049, "Spectral emittance"=0.021365228106035507}, {95.20479999999999, "Spectral emittance"=0.021282265568833277}, {95.3047, "Spectral emittance"=0.02119970426513761}, {95.4046, "Spectral emittance"=0.021117541875176817}, {95.5045, "Spectral emittance"=0.02103577609476399}, {95.6044, "Spectral emittance"=0.020954404635177924}, {95.7043, "Spectral emittance"=0.020873425223044938}, {95.8042, "Spectral emittance"=0.020792835600221764}, {95.9041, "Spectral emittance"=0.020712633523679407}, {96.00399999999999, "Spectral emittance"=0.020632816765388085}, {96.1039, "Spectral emittance"=0.02055338311220294}, {96.2038, "Spectral emittance"=0.020474330365751033}, {96.30369999999999, "Spectral emittance"=0.02039565634231902}, {96.4036, "Spectral emittance"=0.020317358872741914}, {96.5035, "Spectral emittance"=0.020239435802292788}, {96.6034, "Spectral emittance"=0.020161884990573392}, {96.7033, "Spectral emittance"=0.020084704311405733}, {96.8032, "Spectral emittance"=0.02000789165272448}, {96.9031, "Spectral emittance"=0.019931444916470437}, {97.003, "Spectral emittance"=0.01985536201848476}, {97.10289999999999, "Spectral emittance"=0.01977964088840418}, {97.2028, "Spectral emittance"=0.01970427946955701}, {97.3027, "Spectral emittance"=0.019629275718860157}, {97.40259999999999, "Spectral emittance"=0.019554627606716918}, {97.5025, "Spectral emittance"=0.019480333116915563}, {97.6024, "Spectral emittance"=0.019406390246528994}, {97.7023, "Spectral emittance"=0.019332797005815062}, {97.8022, "Spectral emittance"=0.019259551418117696}, {97.90209999999999, "Spectral emittance"=0.019186651519769057}, {98.002, "Spectral emittance"=0.019114095359992308}, {98.1019, "Spectral emittance"=0.019041881000805377}, {98.20179999999999, "Spectral emittance"=0.018970006516925302}, {98.3017, "Spectral emittance"=0.018898469995673628}, {98.4016, "Spectral emittance"=0.018827269536882435}, {98.5015, "Spectral emittance"=0.018756403252801153}, {98.6014, "Spectral emittance"=0.01868586926800422}, {98.7013, "Spectral emittance"=0.018615665719299512}, {98.8012, "Spectral emittance"=0.018545790755637472}, {98.9011, "Spectral emittance"=0.018476242538020986}, {99.00099999999999, "Spectral emittance"=0.01840701923941615}, {99.1009, "Spectral emittance"=0.018338119044663575}, {99.2008, "Spectral emittance"=0.018269540150390586}, {99.30069999999999, "Spectral emittance"=0.018201280764924086}, {99.4006, "Spectral emittance"=0.018133339108204145}, {99.5005, "Spectral emittance"=0.01806571341169828}, {99.6004, "Spectral emittance"=0.017998401918316552}, {99.7003, "Spectral emittance"=0.01793140288232715}, {99.8002, "Spectral emittance"=0.017864714569272966}, {99.9001, "Spectral emittance"=0.01779833525588853}]}, ...(2 in all)]
  in  "stop":bool
  in  "Surface Temperature (K)":dbl=5778.0 step=1000.0
  in  "Max":dbl=100.0
  in  "Min":dbl=0.1
  # "Sun"
  # "Earth"
  # "* At Earth's mean distance from Sun per average surface area of Earth"
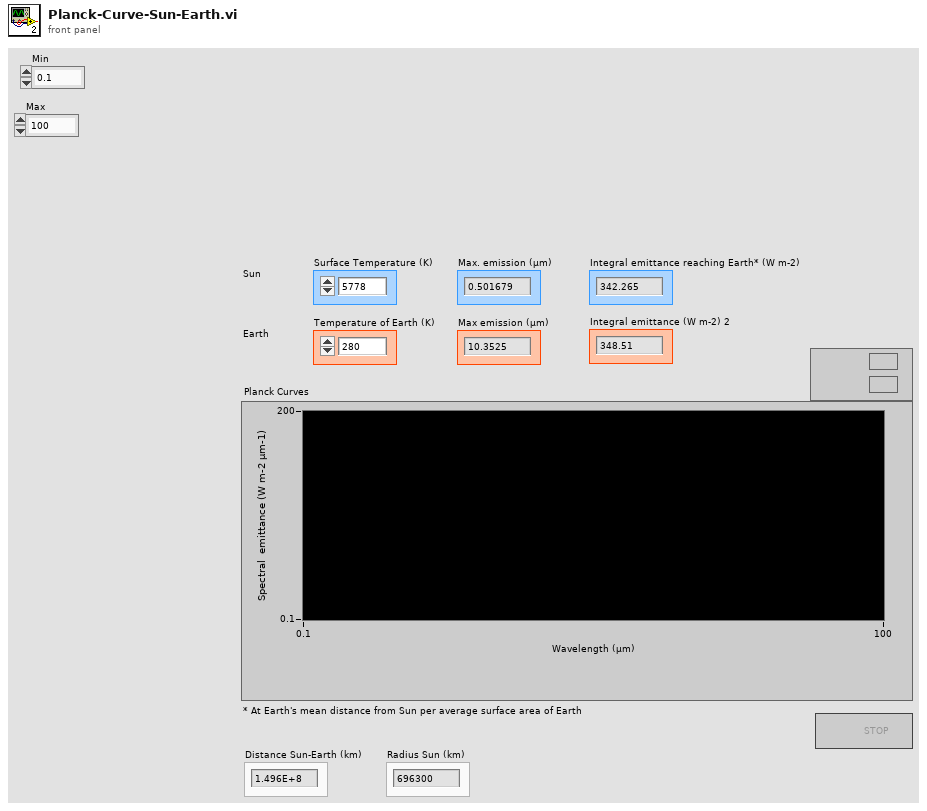
[diagram p1: front panel]
types:
  T1 = cluster{cluster{dbl, "Spectral emittance":dbl[unit]}[]}[]
  T2 = cluster{cluster{dbl, "Spectral emittance":dbl[unit]}[]}
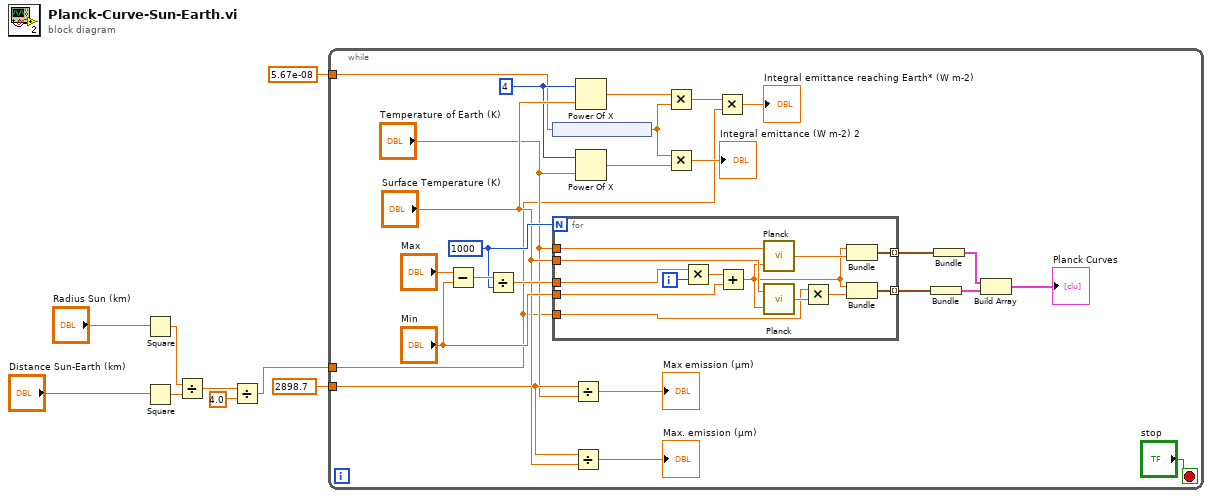
[diagram p0: block diagram]
diagram:
  n1 = Square(x="Radius Sun (km)") -> (x^2=w5:dbl[unit])
  n2 = Square(x="Distance Sun-Earth (km)") -> (x^2=w4:dbl[unit])
  n3 = Divide(x=w5, y=w4) -> (x/y=w3:dbl)
  n4 = Divide(x=w3, y=4.0) -> (x/y=w1:dbl)
  n5 = while {
    tunnel: 2898.7 -> [w26]
    tunnel: 5.67e-08 -> [w14]
    tunnel: w1 -> [w10]
    stop <- "stop" stop-if-true
    w18 = 4
    w32 = 1000 ("dimension size")
    n6 = Subtract(x="Max", y="Min") -> (x-y=w33:dbl)
    n7 = Divide(x=w33, y=w32) -> (x/y=w31:dbl)
    n8 = node(w14) -> (w15:dbl[unit])
    n9 = for {
      N: w32 -> [_]
      tunnel: w31 -> [w46]
      tunnel: "Min" -> [w44]
      tunnel: "Surface Temperature (K)" -> [w43]
      tunnel: "Temperature of Earth (K)" -> [w42]
      tunnel: [w39] -> w25 mode=indexing
      tunnel: [w36] -> w24 mode=indexing
      tunnel: w10 -> [w35]
      i -> [w47]
      n10 = Multiply(x=w46, y=w47) -> (x*y=w45:dbl)
      n11 = Add(x=w45, y=w44) -> (x+y=w38:dbl)
      n12 = call "Planck.vi"("Wavelength (µm)"=w38, "Temperature"=w42) -> ("Spectral emittance"=w40:dbl[unit])
      n13 = call "Planck.vi"("Wavelength (µm)"=w38, "Temperature"=w43) -> ("Spectral emittance"=w41:dbl[unit])
      n14 = Multiply(x=w35, y=w41) -> (x*y=w37:dbl[unit])
      n15 = Bundle(w38, "Spectral emittance"=w40) -> (w39:cluster{dbl, "Spectral emittance":dbl[unit]})  [unwired: 1 in]
      n16 = Bundle(w38, w37) -> (w36:cluster{dbl, dbl[unit]})  [unwired: 1 in]
    }
    n17 = Divide(x=w26, y="Temperature of Earth (K)") -> (x/y=→"Max emission (µm)":dbl)
    n18 = Divide(x=w26, y="Surface Temperature (K)") -> (x/y=→"Max. emission (µm)":dbl)
    n19 = Power Of X(1:"Surface Temperature (K)", 2:w18) -> (0:w19:dbl)
    n20 = Power Of X(1:"Temperature of Earth (K)", 2:w18) -> (0:w16:dbl)
    n21 = Multiply(x=w19, y=w15) -> (x*y=w11:dbl[unit])
    n22 = Multiply(x=w15, y=w16) -> (x*y=→"Integral emittance (W m-2) 2":dbl[unit])
    n23 = Multiply(x=w11, y=w10) -> (x*y=→"Integral emittance reaching Earth* (W m-2)":dbl[unit])
    n24 = Bundle "Bundle"(w24) -> (w23:cluster{cluster{dbl, dbl[unit]}[]})  [unwired: 1 in]
    n25 = Bundle(w25) -> (w22:T2)  [unwired: 1 in]
    n26 = Build Array "Build Array"(w22, w23) -> (→"Planck Curves":T1)
  }
